vi "4a.vi"() -> ()   [LabVIEW 2015]
panel:
  in  "physical channels 2":tag="Dev1/ai0:2"
  in  "Sampling rate 2":dbl=10000.0
  in  "# of samples/channel 2":i32=1000
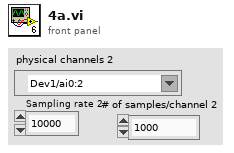
[diagram p1: front panel]
types:
  T1 = enum16{"open", "replace", "create", "open or create", "replace or create", "replace or create with confirmation"}
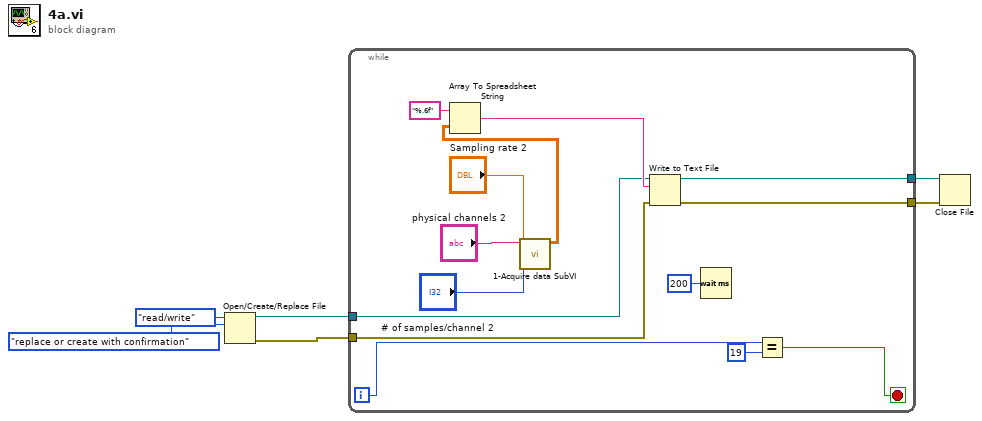
[diagram p0: block diagram]
diagram:
  n1 = Open/Create/Replace File(operation (0:open)=T1."replace or create with confirmation", access (0:read/write)=enum16{"read/write", "read-only", "write-only"}."read/write") -> (refnum out=w2:refnum<file>, error out=w1:errorcluster)  [unwired: 4 in, 1 out]
  n2 = while {
    tunnel: [w14] -> w6
    tunnel: [w13] -> w5
    tunnel: w2 -> [w12]
    tunnel: w1 -> [w11]
    i -> [w19]
    stop <- w17 stop-if-true
    n3 = call "1-Acquire data SubVI.vi"("# of samples/channel"="# of samples/channel 2", "Sampling rate"="Sampling rate 2", "physical channels"="physical channels 2") -> ("data"=w7:dbl[][])  [unwired: 8 in]
    n4 = Array To Spreadsheet String(array=w7, 3:"%.6f" ("format string")) -> (spreadsheet string=w15:string)  [unwired: 1 in]
    n5 = Write to Text File(file (use dialog)=w12, text=w15, error in=w11) -> (refnum out=w13:refnum<file>, error out=w14:errorcluster)  [unwired: 1 in, 1 out]
    n6 = Wait (ms)(milliseconds to wait=u32 200) -> ()  [unwired: 1 out]
    n7 = Equal?(x=w19, y=19) -> (x = y?=w17:bool)
  }
  n8 = Close File(refnum=w5, error in=w6) -> ()  [unwired: 2 out]
